vi "Reset Device.vi"(8 "error in (no error)":errorcluster, 11 "IVI_DMM in":refnum<class "IVI_DMM.lvclass">) -> (0 "error out":errorcluster, 3 "IVI_DMM out":refnum<class "IVI_DMM.lvclass">)   [LabVIEW 2013, in "IVI-DMM.lvlib" / "IVI_DMM.lvclass"]
doc: "Perform reset of device."
uses:
  IVI_DMM.lvclass
  IVI_DMM.lvclass/IVI_DMM.ctl
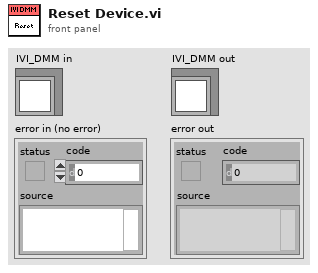
[diagram p1: front panel]
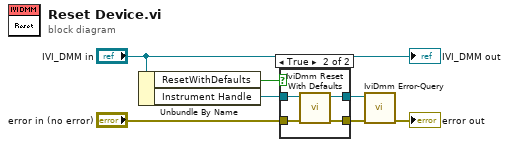
[diagram p0: block diagram]
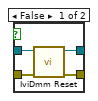
[diagram p2: hidden frame]
diagram:
  n1 = Unbundle By Name("IVI_DMM in") -> ("ResetWithDefaults"=w4:bool, "Instrument Handle"=w6:refnum<k15>)
  n2 = case shown="True" w4 {
    tunnel: w6 -> [w10 w15]
    tunnel: "error in (no error)" -> [w11 w14]
    tunnel: [w9 w13] -> w3
    tunnel: [w8 w12] -> w2
    frame False {
      n3 = call <vilib>:"IviDmm Reset.vi"("error in (no error)"=w11, "instrument handle"=w10) -> ("error out"=w9:errorcluster, "instrument handle out"=w8:refnum<k15>)  [unwired: 8 in]
    }
    frame True {
      n4 = call <vilib>:"IviDmm Reset With Defaults.vi"("error in (no error)"=w14, "instrument handle"=w15) -> ("error out"=w13:errorcluster, "instrument handle out"=w12:refnum<k15>)  [unwired: 8 in]
    }
  }
  n5 = call <vilib>:"IviDmm Error-Query.vi"("error in (no error)"=w3, "instrument handle"=w2) -> ("error out"=→"error out":errorcluster)  [unwired: 6 in, 3 out]
  "IVI_DMM out" <- "IVI_DMM in"
